vi "Motor Move XYZ-AOL Zstack.vi"(8 "error in (no error)":errorcluster, 9 "Zplane in":i32, 10 "AOL_Globals":T1={"Imaging Protocol"=enum."AOL Z-Stack", "Number of POI"=0, "Number of Miniscans"=0, "Number of Trials"=0, "Number of Cycles "=0, "# Averaged Frames"=0, "Laser power (%)"=0, "Pockels"=0.0, "Acquisition Length (sec)"=0.0, "Fill time (us)"=0.0, "POI Dwell time (us)"=0.0, "Miniscan Dwell time per pixel (us)"=0.0, "PMT 1"=0.0, "PMT 2"=0.0, "Back Apperture"=200.0, "Frame Size"=0, "Center Frequency"=0.0, "Field of View"=0.0, "DwellTime (us)"=0.0, "Wavelength (nm)"=0.0, "Zoom"=0.0, "AOL Z"=0.0, "AOL Mode"=enum."Raster", "GridXY"=0.0, "GridZ"=0.0, "TriggerPeriod (sec)"=0.0, "Number of Pixels in Miniscan"=0, "Experiment folder path"=path "", "X centre"=0.0, "Y centre"=0.0, "Angle (degrees)"=0.0, "Plane Mode"=0, "Threshold"=[], "Regenerate Chirps"=FALSE, "Rectangle ROI length (pixels)"=0, "Rectangle ROI height (pixels)"=0, "AOD fill"=0, "Samples Wait after Trigger"=0, "StartUp Delay"=0, "Slip Cycle"=163840, "Add Cycle"=FALSE} {"Plane Mode" items=["XY Plane"]; "Frame Size" items=["100X100"=100, "128X128"=128, "200X200"=200, "256X256"=256, "512X512"=512, "1024x1024"=1024, "2048x2048"=2048]; "Back Apperture" format="%#.6g"; "Pockels" format="%#.6g"; "PMT 2" format="%#.6g"; "PMT 1" format="%#.6g"; "Angle (degrees)" format="%#.6g"; "POI Dwell time (us)" format="%#.6g"}) -> (0 "error out":errorcluster)   [LabVIEW 2013]
uses:
  Typedefs/Controls/AOL_Globals.ctl
  Typedefs/Imaging Protocols enum.ctl
  Typedefs/Frame Size.ctl
  Typedefs/AOL modes.ctl
  Typedefs/Plane Mode.ctl
  Typedefs/Read Write Enum.ctl
  Global Variables/General Globals.vi
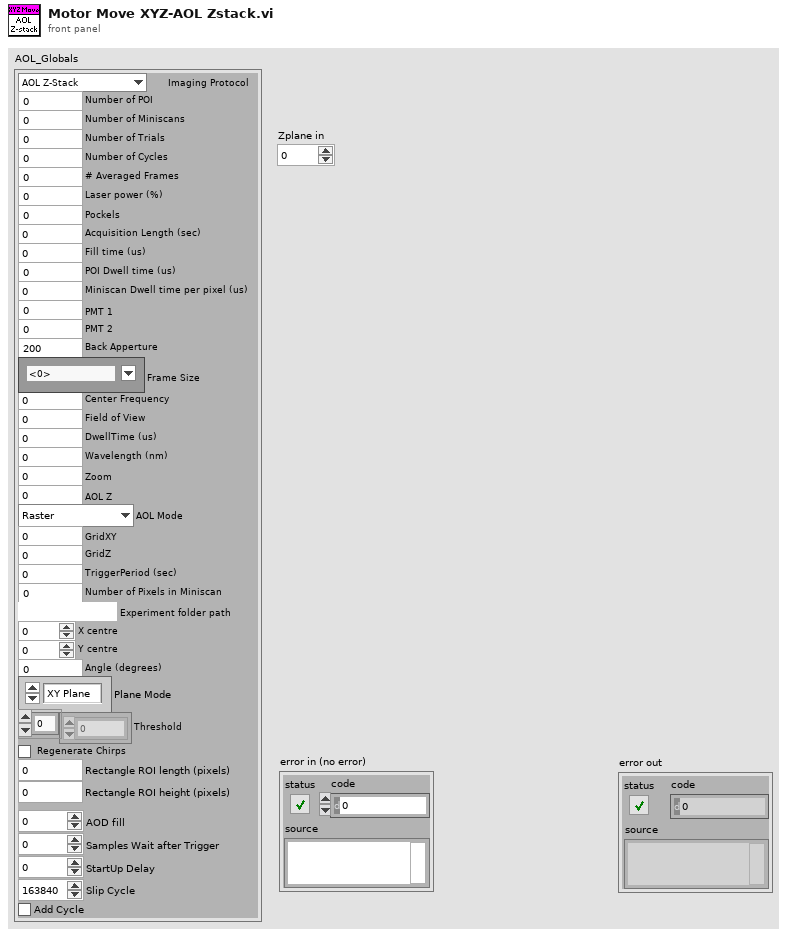
[diagram p1: front panel]
types:
  T1 = typedef "AOL_Globals.ctl" = cluster{"Imaging Protocol":T2, "Number of POI":u16, "Number of Miniscans":u16, "Number of Trials":u16, "Number of Cycles ":u64, "# Averaged Frames":u16, "Laser power (%)":u8, "Pockels":dbl, "Acquisition Length (sec)":dbl, "Fill time (us)":dbl, "POI Dwell time (us)":dbl, "Miniscan Dwell time per pixel (us)":dbl, "PMT 1":dbl, "PMT 2":dbl, "Back Apperture":dbl, "Frame Size":T3, "Center Frequency":dbl, "Field of View":dbl, "DwellTime (us)":dbl, "Wavelength (nm)":dbl, "Zoom":dbl, "AOL Z":dbl, "AOL Mode":T4, "GridXY":dbl, "GridZ":dbl, "TriggerPeriod (sec)":dbl, "Number of Pixels in Miniscan":u16, "Experiment folder path":path, "X centre":dbl, "Y centre":dbl, "Angle (degrees)":dbl, "Plane Mode":T5, "Threshold":u16[], "Regenerate Chirps":bool, "Rectangle ROI length (pixels)":u16, "Rectangle ROI height (pixels)":u16, "AOD fill":u16, "Samples Wait after Trigger":u16, "StartUp Delay":i32, "Slip Cycle":u32, "Add Cycle":bool}
  T2 = typedef "Imaging Protocols enum.ctl" = enum16{"AOL Z-Stack", "Motor Z Stack", "Functional Acquisition", "Single Plane Acquisition", "Volume Acquisition", "Live Imaging", "Live Plane Imaging", "Live Volume Imaging"}
  T3 = typedef "Frame Size.ctl" = u16
  T4 = typedef "AOL modes.ctl" = enum16{"Raster", "Structural", "Pointing", "Mini Scan", "Alignment"}
  T5 = typedef "Plane Mode.ctl" = u16
  T6 = typedef "Read Write Enum.ctl" = enum16{"Read", "Write"}
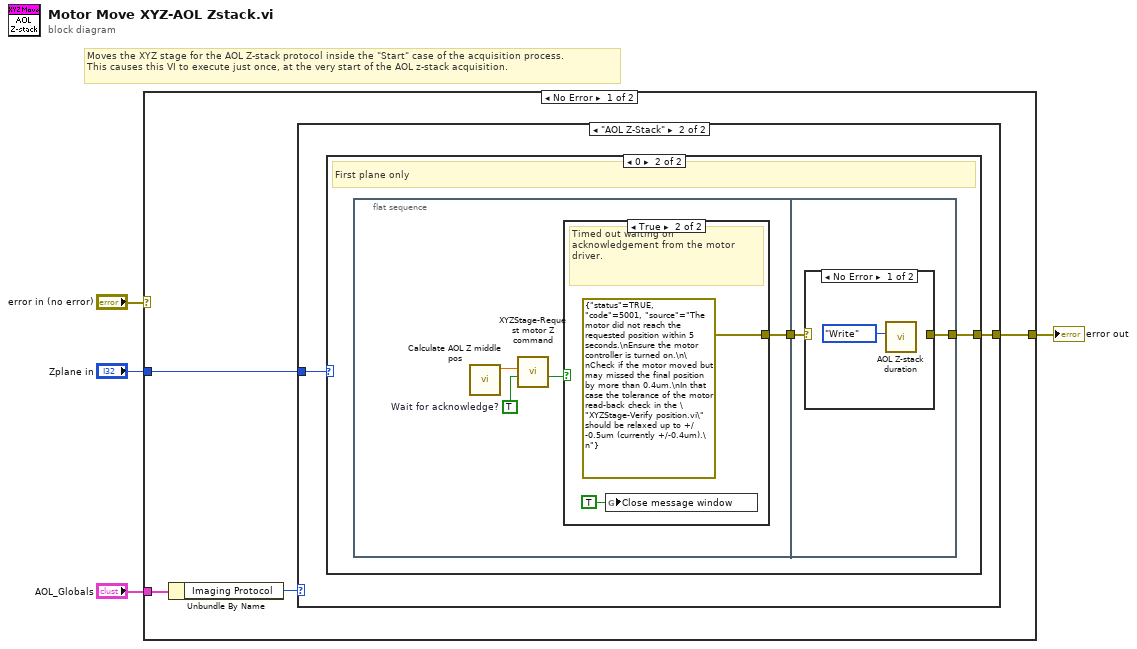
[diagram p0: block diagram]
diagram:
  # "Moves the XYZ stage for the AOL Z-stack protocol inside the \"Start\" case of the acquisition process.\nThis causes this VI to execute just once, at the very start of the AOL z-stack acquisition."
  n1 = case shown="No Error" "error in (no error)" {
    selector: "error in (no error)" -> [_ w23]
    tunnel: [w5 w23] -> w3
    tunnel: "AOL_Globals" -> [w7 _]
    tunnel: "Zplane in" -> [w6 _]
    frame No Error {
      n2 = Unbundle By Name(w7) -> ("Imaging Protocol"=w8:T2)
      n3 = case shown="\"AOL Z-Stack\"" w8 {
        tunnel: w6 -> [_ w10]
        tunnel: [_ w9] -> w5
        frame Default {
        }
        frame "AOL Z-Stack" {
          n4 = case shown="0" w10 {
            tunnel: [_ w11] -> w9
            frame Default {
            }
            frame 0 {
              # "First plane only"
              n5 = flat-sequence {
                tunnel: [w13] -> w12
                tunnel: w12 -> [w20]
                tunnel: [w19] -> w11
                frame #0 {
                  w15 = TRUE  # Wait for acknowledge?
                  n6 = call "Calculate AOL Z middle pos.vi"() -> ("AOL Z-stack middle position"=w16:dbl)  [unwired: 11 in]
                  n7 = call "XYZStage-Request motor Z command.vi"("Wait for acknowledge?"=w15, "Motor Z"=w16) -> ("Timed out while waiting for acknowledgement"=w14:bool)  [unwired: 7 in, 2 out]
                  n8 = case shown="True" w14 {
                    tunnel: [_ errorcluster {"status"=TRUE, "code"=5001, "source"="The motor did not reach the requested position within 5 seconds.\nEnsure the motor controller is turned on.\n\nCheck if the motor moved but may missed the final position by more than 0.4um.\nIn that case the tolerance of the motor read-back check in the \"XYZStage-Verify position.vi\" should be relaxed up to +/-0.5um (currently +/-0.4um).\n"} ("error IO")] -> w13
                    frame False {
                    }
                    frame True {
                      # "Timed out waiting on acknowledgement from the motor driver."
                      n9 = global write "General Globals.vi" "Close message window"(TRUE ("Close message window")) -> ()
                    }
                  }
                }
                frame #1 {
                  n10 = case shown="No Error" w20 {
                    selector: w20 -> [_ w22]
                    tunnel: [_ w22] -> w19
                    frame No Error {
                      n11 = call "AOL Z-stack duration.vi"("Function"=Read_Write_Enum."Write") -> ()  [unwired: 10 in, 1 out]
                    }
                    frame Error {
                    }
                  }
                }
              }
            }
          }
        }
      }
    }
    frame Error {
    }
  }
  "error out" <- w3
